vi "Segway - Segue objeto.vi"() -> ()   [LabVIEW 2016]
uses:
  <vilib>/NXT/Block Support/NXT_InputPort.ctl
  <vilib>/NXT/Subs/MotorOutput.ctl
  <vilib>/NXT/Block Support/NXT_TimerIndex.ctl
  <vilib>/NXT/Block Support/NXT_OutputPort.ctl
  <vilib>/NXT/Dual Mode Library/Waits/Wait_Num.vi
  <vilib>/NXT/Dual Mode Library/Sensors/EV3_Gyro_Reset.vi
  <vilib>/NXT/Dual Mode Library/Motors/ResetMotor.vi
  <vilib>/NXT/Dual Mode Library/Sensors/EV3_Color_Reflect.vi
  <vilib>/NXT/Dual Mode Library/Display/drawNumber.vi
  <vilib>/NXT/Dual Mode Library/Sensors/EV3_Gyro_Rate.vi
  <vilib>/NXT/Dual Mode Library/Motors/Rotation.vi
  <vilib>/NXT/NXTIO Xnodes/NXTIONodeSubVIs/NXTMoveMotors.vi
  <vilib>/NXT/NXTIO Xnodes/AddressXNode/NXTIOAddress.xnode
  <vilib>/NXT/NXTIO Xnodes/NXTIOXNode/NXTIO.xnode
  <vilib>/NXT/Subs/LVHSConnector.ctl
  <vilib>/NXT/LegoClasses/BrickReference/BrickReference.lvclass
panel:
  in  "stop":bool
  out "e":dbl
  out "Waveform Chart 2":dbl(graph)
  out "b":dbl
  out "a":dbl
  in  "dt_program_flow":dbl
  out "dt":dbl
  out "timer_time":dbl
  out "EncSum":dbl
  out "VelAngRoda2":dbl(graph)
  out "PosAngRoda2":dbl(graph)
  out "PosAngCorpo2":dbl(graph)
  out "VelAngCorpo2":dbl(graph)
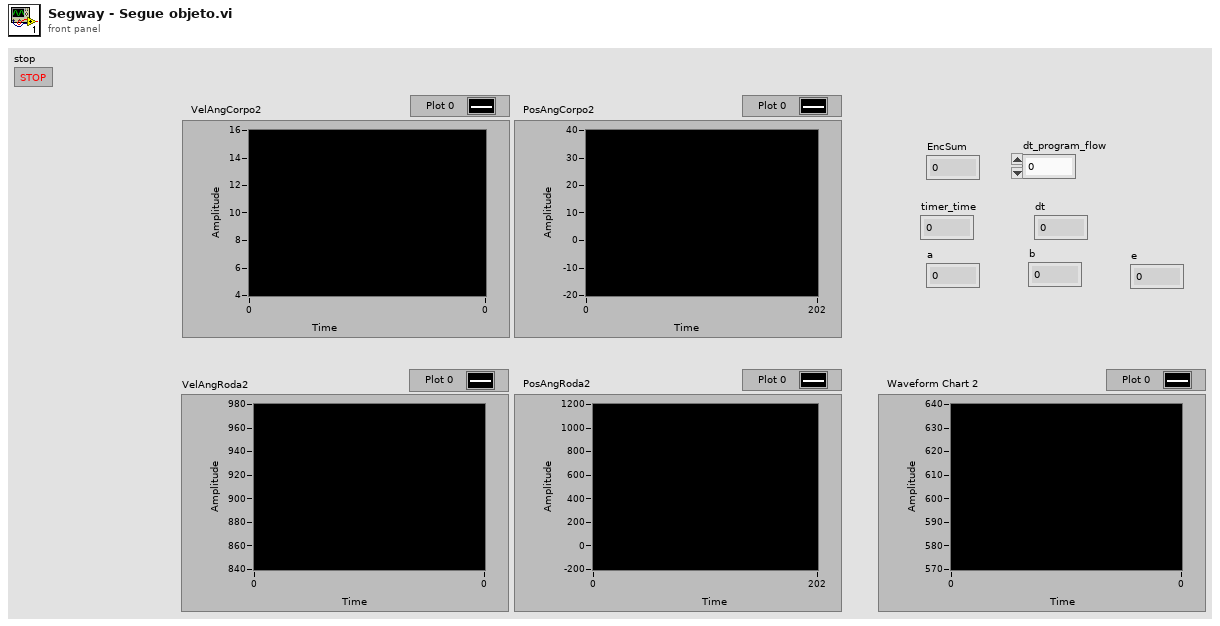
[diagram p1: front panel]
types:
  T1 = typedef "NXT_TimerIndex.ctl" = u8
  T2 = typedef "MotorOutput.ctl" = u8
  T3 = typedef "NXT_InputPort.ctl" = u32
  T4 = typedef "LVHSConnector.ctl" = refnum<class "BrickReference.lvclass">
  T5 = typedef "NXT_OutputPort.ctl" = u8
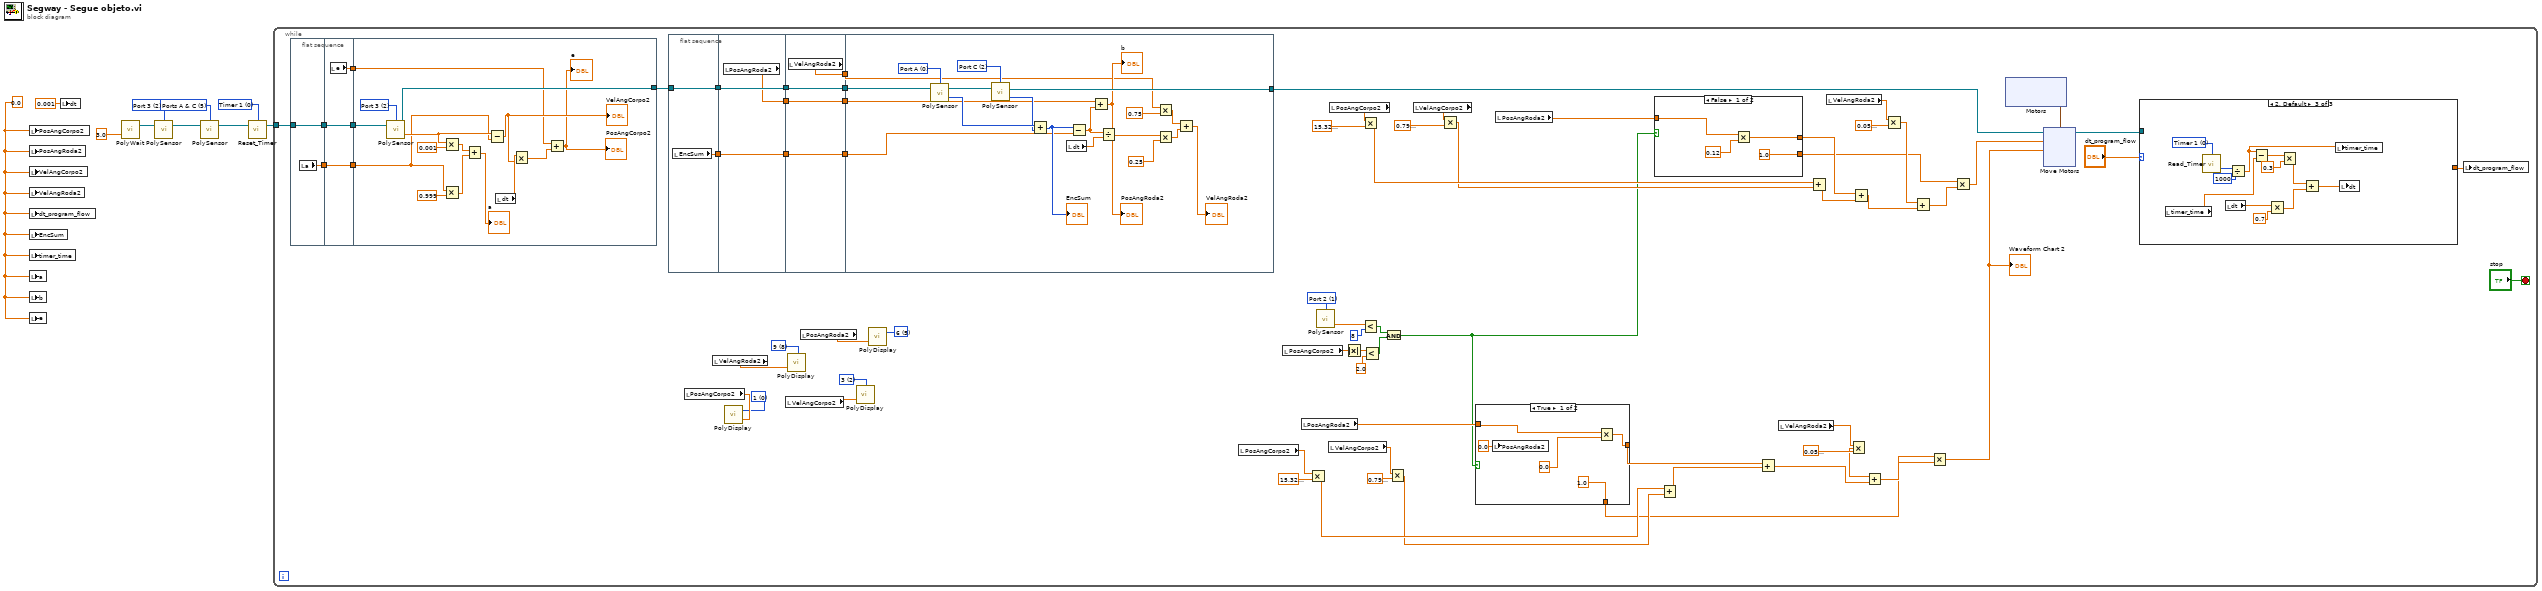
[diagram p0: block diagram]
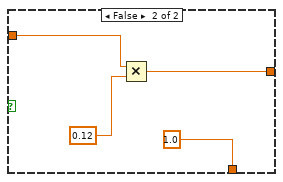
[diagram p2: hidden frame]
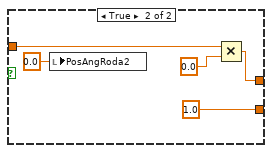
[diagram p3: hidden frame]
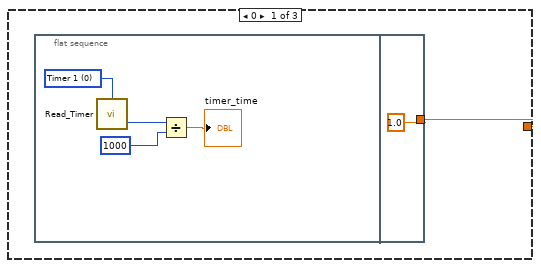
[diagram p4: hidden frame]
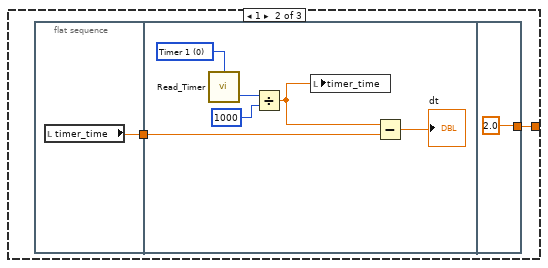
[diagram p5: hidden frame]
diagram:
  w3 = T1 0 items=["Timer 1", "Timer 2", "Timer 3"] ("Timer (Timer 1)")
  w8 = T2 5 items=["Port A"=0, "Port B"=1, "Port C"=2, "Ports A & B"=4, "Ports A & C"=5, "Ports B & C"=6, "All Ports"=3] ("Port (All Ports)")
  w9 = T3 2 items=["Port 1", "Port 2", "Port 3", "Port 4"] ("Port (Port 1)")
  w5 = 0.0 ("PosAngCorpo2")
  n1 = local write "PosAngCorpo2"(w5) -> ()
  n2 = local write "PosAngRoda2"(w5) -> ()
  n3 = local write "VelAngCorpo2"(w5) -> ()
  n4 = local write "VelAngRoda2"(w5) -> ()
  n5 = local write "dt_program_flow"(w5) -> ()
  n6 = local write "EncSum"(w5) -> ()
  n7 = local write "timer_time"(w5) -> ()
  n8 = local write "a"(w5) -> ()
  n9 = local write "b"(w5) -> ()
  n10 = local write "e"(w5) -> ()
  n11 = local write "dt"(0.001 ("dt")) -> ()
  n12 = call-poly <vilib>:"PolyWait.vi"("Time (1 sec)"=sgl 3.0) -> ("NXT/EV3"=w4:T4)  [unwired: 3 in]
  n13 = call-poly <vilib>:"PolySensor.vi"("NXT/EV3"=w4, "Port (Port 1)"=w9) -> ("NXT/EV3"=w7:T4)  [unwired: 2 in]
  n14 = call-poly <vilib>:"PolySensor.vi"("NXT/EV3"=w7, "Port (All Ports)"=w8) -> ("NXT/EV3"=w1:T4)  [unwired: 2 in]
  n15 = call <vilib>:"Reset_Timer.vi"("NXT/EV3"=w1, "Timer (Timer 1)"=w3) -> ("NXT/EV3"=w2:T4)  [unwired: 2 in]
  n16 = while {
    tunnel: w2 -> [w69]
    stop <- "stop" stop-if-true
    w28 = T3 1 items=["Port 1", "Port 2", "Port 3", "Port 4"] ("Port (Port 4)")
    w44 = i16 5 items=["1", "2", "3", "4", "5", "6", "7", "8", "9", "10", "11", "12"] ("Line")
    w45 = i16 8 items=["1", "2", "3", "4", "5", "6", "7", "8", "9", "10", "11", "12"] ("Line")
    w46 = i16 2 items=["1", "2", "3", "4", "5", "6", "7", "8", "9", "10", "11", "12"] ("Line")
    w48 = i16 0 items=["1", "2", "3", "4", "5", "6", "7", "8", "9", "10", "11", "12"] ("Line")
    n17 = flat-sequence {
      tunnel: w69 -> [w130]
      tunnel: [w130] -> w63
      tunnel: [w129] -> w61
      tunnel: w63 -> [w133]
      tunnel: [w133] -> w62
      tunnel: w61 -> [w132]
      tunnel: [w132] -> w60
      tunnel: [w131] -> w59
      tunnel: [w140] -> w72
      tunnel: w62 -> [w136]
      tunnel: w60 -> [w135]
      tunnel: w59 -> [w134]
      frame #0 {
        n18 = local read "a"() -> (w129:dbl)
      }
      frame #1 {
        n19 = local read "e"() -> (w131:dbl)
      }
      frame #2 {
        w144 = T3 2 items=["Port 1", "Port 2", "Port 3", "Port 4"] ("Port (Port 1)")
        n20 = call-poly <vilib>:"PolySensor.vi"("NXT/EV3"=w136, "Port (Port 1)"=w144) -> ("Degrees/Second"=w143:sgl, "NXT/EV3"=w140:T4)  [unwired: 1 in]
        n21 = Multiply(x=w143, y=0.001) -> (x*y=w146:dbl)
        n22 = Multiply(x=w135, y=0.999) -> (x*y=w139:dbl)
        n23 = Add(x=w146, y=w139) -> (x+y=→"a":dbl)
        n24 = Subtract(x=w143, y=w135) -> (x-y=w141:dbl)
        "VelAngCorpo2" <- w141
        n25 = local read "dt"() -> (w142:dbl)
        n26 = Multiply(x=w142, y=w141) -> (x*y=w145:dbl)
        n27 = Add(x=w134, y=w145) -> (x+y=→"PosAngCorpo2" →"e":dbl)
      }
    }
    n28 = flat-sequence {
      tunnel: w72 -> [w101]
      tunnel: [w101] -> w58
      tunnel: [w100] -> w57
      tunnel: w58 -> [w104]
      tunnel: [w104] -> w56
      tunnel: w57 -> [w103]
      tunnel: [w103] -> w54
      tunnel: [w102] -> w51
      tunnel: w56 -> [w108]
      tunnel: [w108] -> w55
      tunnel: w54 -> [w107]
      tunnel: [w107] -> w53
      tunnel: [w106] -> w52
      tunnel: w51 -> [w105]
      tunnel: [w105] -> w50
      tunnel: w55 -> [w117]
      tunnel: [w115] -> w71
      tunnel: w53 -> [w111]
      tunnel: w52 -> [w110]
      tunnel: w50 -> [w109]
      frame #0 {
        n29 = local read "EncSum"() -> (w100:dbl)
      }
      frame #1 {
        n30 = local read "PosAngRoda2"() -> (w102:dbl)
      }
      frame #2 {
        n31 = local read "VelAngRoda2"() -> (w106:dbl)
      }
      frame #3 {
        w119 = T5 2 items=["Port A", "Port B", "Port C", "Port D"] ("Port (Port A)")
        w122 = T5 0 items=["Port A", "Port B", "Port C", "Port D"] ("Port (Port A)")
        n32 = call-poly <vilib>:"PolySensor.vi"("NXT/EV3"=w117, "Port (Port A)"=w122) -> ("Angle of Rotation"=w121:i32, "NXT/EV3"=w116:T4)  [unwired: 1 in]
        n33 = call-poly <vilib>:"PolySensor.vi"("NXT/EV3"=w116, "Port (Port A)"=w119) -> ("Angle of Rotation"=w118:i32, "NXT/EV3"=w115:T4)  [unwired: 1 in]
        n34 = Add(x=w121, y=w118) -> (x+y=w128:i32)
        "EncSum" <- w128
        n35 = local read "dt"() -> (w120:dbl)
        n36 = Subtract(x=w128, y=w111) -> (x-y=w127:dbl)
        n37 = Add(x=w109, y=w127) -> (x+y=→"PosAngRoda2" →"b":dbl)
        n38 = Divide(x=w127, y=w120) -> (x/y=w123:dbl)
        n39 = Multiply(x=w110, y=0.75) -> (x*y=w113:dbl)
        n40 = Multiply(x=w123, y=sgl 0.25) -> (x*y=w125:dbl)
        n41 = Add(x=w113, y=w125) -> (x+y=→"VelAngRoda2":dbl)
      }
    }
    n42 = local read "PosAngCorpo2"() -> (w49:dbl)
    n43 = local read "VelAngRoda2"() -> (w42:dbl)
    n44 = call-poly <vilib>:"PolyDisplay.vi"("number"=w49, "Line"=w48) -> ()  [unwired: 2 in, 1 out]
    n45 = local read "VelAngCorpo2"() -> (w47:dbl)
    n46 = call-poly <vilib>:"PolyDisplay.vi"("number"=w42, "Line"=w45) -> ()  [unwired: 2 in, 1 out]
    n47 = local read "PosAngRoda2"() -> (w43:dbl)
    n48 = call-poly <vilib>:"PolyDisplay.vi"("number"=w47, "Line"=w46) -> ()  [unwired: 2 in, 1 out]
    n49 = call-poly <vilib>:"PolyDisplay.vi"("number"=w43, "Line"=w44) -> ()  [unwired: 2 in, 1 out]
    n50 = local read "PosAngCorpo2"() -> (w19:dbl)
    n51 = local read "PosAngCorpo2"() -> (w12:dbl)
    n52 = local read "PosAngRoda2"() -> (w17:dbl)
    n53 = Multiply(x=w19, y=sgl 15.33) -> (x*y=w33:dbl)
    n54 = call-poly <vilib>:"PolySensor.vi"("Port (Port 1)"=w28) -> ("Scaled Value"=w26:sgl)  [unwired: 2 in, 1 out]
    n55 = local read "VelAngCorpo2"() -> (w20:dbl)
    n56 = local read "PosAngCorpo2"() -> (w75:dbl)
    n57 = Absolute Value(x=w12) -> (abs(x)=w21:dbl)
    n58 = Multiply(x=w75, y=sgl 15.33) -> (x*y=w68:dbl)
    n59 = Less?(x=w26, y=i16 8) -> (x < y?=w24:bool)
    n60 = Less?(x=w21, y=2.0) -> (x < y?=w23:bool)
    n61 = And(x=w24, y=w23) -> (x .and. y?=w11:bool)
    n62 = Multiply(x=w20, y=sgl 0.79) -> (x*y=w32:dbl)
    n63 = local read "VelAngCorpo2"() -> (w74:dbl)
    n64 = Multiply(x=w74, y=sgl 0.79) -> (x*y=w67:dbl)
    n65 = case shown="True" w11 {
      tunnel: w17 -> [w84 w89]
      tunnel: [w83 w88] -> w16
      tunnel: [1.0 1.0 ("y")] -> w15
      frame True {
        n66 = local write "PosAngRoda2"(0.0) -> ()
        n67 = Multiply(x=w84, y=0.0) -> (x*y=w83:dbl)
      }
      frame False {
        n68 = Multiply(x=w89, y=0.12) -> (x*y=w88:dbl)
      }
    }
    n69 = local read "PosAngRoda2"() -> (w40:dbl)
    n70 = case shown="False" w11 {
      tunnel: w40 -> [w94 w98]
      tunnel: [w92 w97] -> w39
      tunnel: [1.0 ("y") 1.0 ("y")] -> w38
      frame False {
        n71 = Multiply(x=w94, y=0.12) -> (x*y=w92:dbl)
      }
      frame True {
        n72 = local write "PosAngRoda2"(0.0 ("PosAngRoda2")) -> ()
        n73 = Multiply(x=w98, y=0.0) -> (x*y=w97:dbl)
      }
    }
    n74 = Add(x=w33, y=w32) -> (x+y=w31:dbl)
    n75 = Add(x=w16, y=w31) -> (x+y=w30:dbl)
    n76 = local read "VelAngRoda2"() -> (w18:dbl)
    n77 = Add(x=w68, y=w67) -> (x+y=w66:dbl)
    n78 = local read "VelAngRoda2"() -> (w73:dbl)
    n79 = Multiply(x=w18, y=sgl 0.06) -> (x*y=w29:dbl)
    n80 = Add(x=w39, y=w66) -> (x+y=w65:dbl)
    n81 = Add(x=w29, y=w30) -> (x+y=w22:dbl)
    n82 = Multiply(x=w73, y=sgl 0.06) -> (x*y=w64:dbl)
    n83 = Add(x=w64, y=w65) -> (x+y=w37:dbl)
    n84 = Multiply(x=w15, y=w22) -> (x*y=w13:dbl)
    "Waveform Chart 2" <- w13
    n85 = Multiply(x=w38, y=w37) -> (x*y=w14:dbl)
    n86 = xnode "Motors"() -> ("Motor"=w79:cluster{"Port":T5, "Port":T5})
    n87 = xnode "Move Motors"("Power/Speed 2"=w13, "Power/Speed 1"=w14, "Motors"=w79, "NXT/EV3"=w71) -> ("NXT/EV3"=w70:T4)
    n88 = case shown="2, Default" "dt_program_flow" {
      tunnel: [w158 w164 _] -> w81
      tunnel: w70 -> [_ _ _]
      frame 0 {
        n89 = flat-sequence {
          tunnel: [1.0 ("dt_program_flow")] -> w158
          frame #0 {
            w162 = T1 0 items=["Timer 1", "Timer 2", "Timer 3"] ("Timer (Timer 1)")
            n90 = call <vilib>:"Read_Timer.vi"("Timer (Timer 1)"=w162) -> ("Value (msec)"=w159:u32)  [unwired: 2 in, 1 out]
            n91 = Divide(x=w159, y=u32 1000) -> (x/y=→"timer_time":dbl)
          }
          frame #1 {
          }
        }
      }
      frame 1 {
        n92 = flat-sequence {
          tunnel: [w166] -> w165
          tunnel: w165 -> [w172]
          tunnel: [2.0 ("dt_program_flow")] -> w164
          frame #0 {
            n93 = local read "timer_time"() -> (w166:dbl)
          }
          frame #1 {
            w170 = T1 0 items=["Timer 1", "Timer 2", "Timer 3"] ("Timer (Timer 1)")
            n94 = call <vilib>:"Read_Timer.vi"("Timer (Timer 1)"=w170) -> ("Value (msec)"=w169:u32)  [unwired: 2 in, 1 out]
            n95 = Divide(x=w169, y=u32 1000) -> (x/y=w167:dbl)
            n96 = local write "timer_time"(w167) -> ()
            n97 = Subtract(x=w167, y=w172) -> (x-y=→"dt":dbl)
          }
          frame #2 {
          }
        }
      }
      frame 2, Default {
        w177 = T1 0 items=["Timer 1", "Timer 2", "Timer 3"] ("Timer (Timer 1)")
        n98 = local read "timer_time"() -> (w174:dbl)
        n99 = call <vilib>:"Read_Timer.vi"("Timer (Timer 1)"=w177) -> ("Value (msec)"=w176:u32)  [unwired: 2 in, 1 out]
        n100 = local read "dt"() -> (w179:dbl)
        n101 = Divide(x=w176, y=u32 1000) -> (x/y=w184:dbl)
        n102 = Subtract(x=w184, y=w174) -> (x-y=w183:dbl)
        n103 = Multiply(x=w179, y=0.7) -> (x*y=w178:dbl)
        n104 = Multiply(x=w183, y=0.3) -> (x*y=w181:dbl)
        n105 = Add(x=w181, y=w178) -> (x+y=w185:dbl)
        n106 = local write "timer_time"(w184) -> ()
        n107 = local write "dt"(w185) -> ()
      }
    }
    n108 = local write "dt_program_flow"(w81) -> ()
  }
